vi "myRIO.vi"() -> ()   [LabVIEW 2018]
uses:
  <vilib>/NI/STM/SubVIs/MetaDataElement.ctl
  <vilib>/NI/STM/TCP/Write Meta Data (TCP Ref).vi
  <vilib>/NI/STM/TCP/Get Connection Reference (TCP).vi
  <vilib>/NI/STM/TCP/Write Meta Data (TCP Clst).vi
  <vilib>/NI/STM/TCP/Read Message (TCP).vi
  <vilib>/NI/STM/TCP/Write Message (TCP).vi
  <vilib>/NI/STM/NI STM.lvlib
panel:
  in  "stop":bool
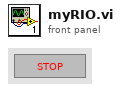
[diagram p1: front panel]
types:
  T1 = typedef "NI STM.lvlib/MetaDataElement.ctl" = string
  T2 = typedef "NI STM.lvlib/TCP Connection Info.ctl" = cluster{"connection ID":refnum<k5>, "meta data":T1[]}
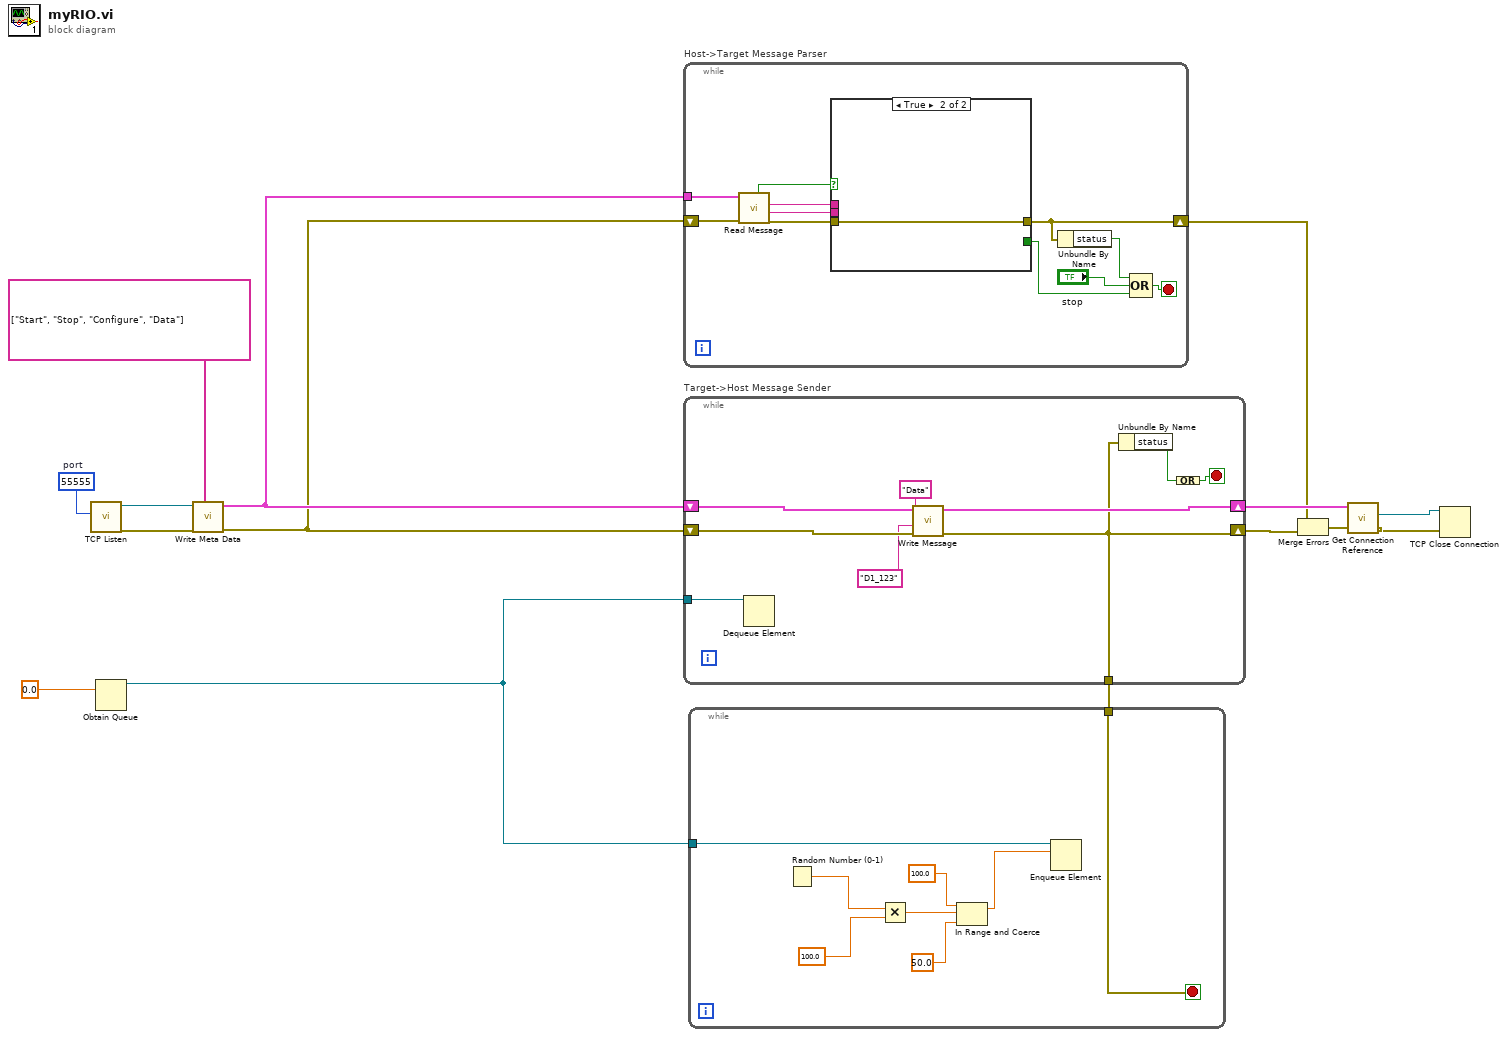
[diagram p0: block diagram]
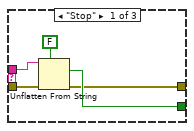
[diagram p3: hidden frame]
diagram:
  w15 = u16 55555  # port
  n1 = call <vilib>:"TCP Listen.vi"("port"=w15) -> ("error out"=w13:errorcluster, "connection ID"=w14:refnum<k5>)  [unwired: 3 in, 6 out]
  n2 = Obtain Queue(element data type=0.0) -> (queue out=w3:refnum<queue>)  [unwired: 4 in, 2 out]
  n3 = call-poly <vilib>:"Write Meta Data.vi"("meta data"=T1[] ["Start", "Stop", "Configure", "Data"], "error in"=w13, "connection ID"=w14) -> ("error out"=w11:errorcluster, "connection info out"=w12:T2)  [unwired: 2 in, 5 out]
  n4 = while "Host->Target Message Parser" {
    tunnel: w12 -> [w26]
    shift-right: [w20] -> w7
    shift-left: w11 -> [w25]
    stop <- w17 stop-if-true
    n5 = call-poly <vilib>:"Read Message.vi"("error in"=w25, "connection info in"=w26) -> ("error out"=w21:errorcluster, "name"=w24:T1, "data string"=w23:string, "timed out?"=w22:bool)  [unwired: 3 in, 3 out]
    n6 = case shown="True" w22 {
      tunnel: w24 -> [w28 _]
      tunnel: w23 -> [w31 _]
      tunnel: w21 -> [w30 w39]
      tunnel: [w29 w39] -> w20
      tunnel: [w27 _] -> w16
      frame False {
        n7 = case shown="Default" w28 {
          tunnel: w31 -> [w35 _ _]
          tunnel: w30 -> [w34 w37 w38]
          tunnel: [w32 w37 w38] -> w29
          tunnel: [w33 _ _] -> w27
          frame "Stop" {
            n8 = Unflatten From String(type=FALSE, binary string=w35, error in (no error)=w34) -> (value=w33:bool, error out=w32:errorcluster)  [unwired: 1 in, 2 out]
          }
          frame "Start" {
          }
          frame Default {
          }
        }
      }
      frame True {
      }
    }
    n9 = Unbundle By Name(w20) -> ("status"=w19:bool)
    n10 = Compound Arithmetic op=OR(w19, "stop", w16) -> (w17:bool)
  }
  n11 = while "Target->Host Message Sender" {
    shift-right: [w41] -> w8
    shift-left: w11 -> [w44]
    shift-right: [w47] -> w10
    shift-left: w12 -> [w48]
    tunnel: w3 -> [w42]
    tunnel: [w41] -> w1
    stop <- w45 stop-if-true
    n12 = Dequeue Element(queue=w42) -> ()  [unwired: 2 in, 4 out]
    n13 = call-poly <vilib>:"Write Message.vi"("error in"=w44, "data"="D1_123", "name"="Data" ("Name"), "connection info in"=w48) -> ("error out"=w41:errorcluster, "connection info out"=w47:T2)  [unwired: 1 in, 5 out]
    n14 = Unbundle By Name(w41) -> ("status"=w46:bool)
    n15 = Compound Arithmetic op=OR(w46) -> (w45:bool)
  }
  n16 = while {
    tunnel: w3 -> [w50]
    tunnel: w1 -> [w49]
    stop <- w49 stop-if-true
    n17 = Random Number (0-1)() -> (number: 0 to 1=w55:dbl)
    n18 = Multiply(x=w55, y=100.0) -> (x*y=w54:dbl)
    n19 = In Range and Coerce(upper limit=100.0, x=w54, lower limit=50.0) -> (coerced(x)=w51:dbl)  [unwired: 1 out]
    n20 = Enqueue Element(queue=w50, element=w51) -> ()  [unwired: 2 in, 3 out]
  }
  n21 = Merge Errors(w7, w8) -> (w6:errorcluster)
  n22 = call-poly <vilib>:"Get Connection Reference.vi"("error in"=w6, "connection info in"=w10) -> ("error out"=w4:errorcluster, "connection ID out"=w9:refnum<k5>)  [unwired: 8 out]
  n23 = TCP Close Connection(connection ID=w9, error in (no error)=w4) -> ()  [unwired: 3 out]
